vi "DSF.Transceiver.UDP.Rx.Read Datagram.vi"(8 "error in (no error)":errorcluster, 10 "Transfer Group Rx parameters":T1={"Transfers Rx"=[], "max size"=548} {"max size" format="%d bytes"; "Transfers Rx"."timeout" format="%d ms"; "Transfers Rx"."max size" format="%d bytes"}, 11 "UDP Transceiver in":refnum<class "DSF.Transceiver.UDP.lvclass">) -> (0 "error out":errorcluster, 1 "data":string, 2 "Transfer index":i32, 3 "UDP Transceiver out":refnum<class "DSF.Transceiver.UDP.lvclass">)   [LabVIEW 2017, in "DSF.Transceiver.UDP.lvlib" / "DSF.Transceiver.UDP.lvclass"]
uses:
  DSF.Transceiver.UDP.lvclass
  DSF.Transceiver.UDP.Parameters.Transfer Group.Rx.ctl
  DSF.Transceiver.UDP.Parameters.Transfer.Rx.ctl
  DSF.Transceiver.UDP.lvclass/DSF.Transceiver.UDP.ctl
  DSF.Transceiver.UDP.Errors.Rx.Unknown Datagram.vi
  <vilib>/NI/Static Error Handling/VIs/Static Error Handling.Source Buffer.Write.String.vi
  <vilib>/NI/Static Error Handling/VIs/Static Error Handling.Source Buffer.Write.Numeric.Scalar.Base10.vi
  <vilib>/NI/Static Error Handling/VIs/Static Error Handling.Source Buffer.Write.Numeric.Scalar.Base10 (U16).vi
  DSF.Transceiver.UDP.Error.Create.vi
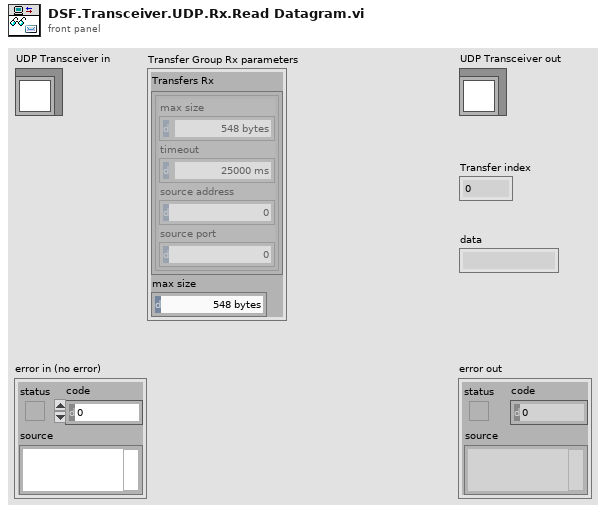
[diagram p1: front panel]
types:
  T1 = typedef "DSF.Transceiver.UDP.lvlib/DSF.Transceiver.UDP.lvclass/DSF.Transceiver.UDP.Parameters.Transfer Group.Rx.ctl" = cluster{"Transfers Rx":T2[], "max size":i32}
  T2 = typedef "DSF.Transceiver.UDP.lvlib/DSF.Transceiver.UDP.lvclass/DSF.Transceiver.UDP.Parameters.Transfer.Rx.ctl" = cluster{"max size":i32, "timeout":i32, "source address":u32, "source port":u16}
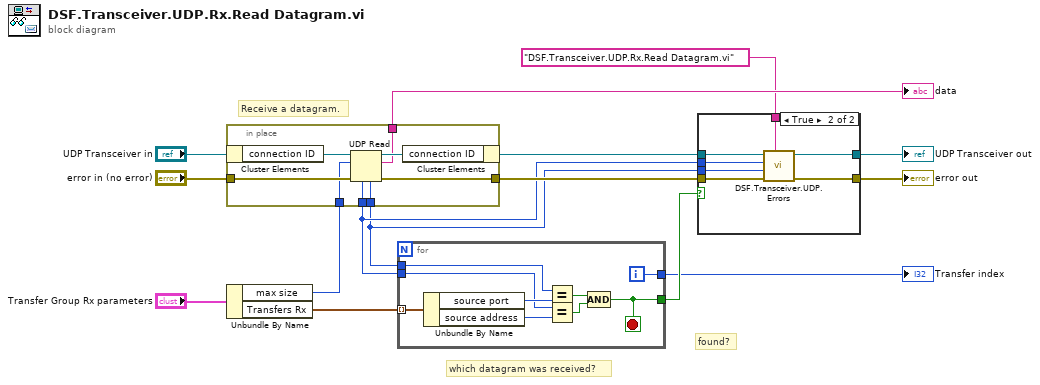
[diagram p0: block diagram]
diagram:
  # "found?"
  # "Receive a datagram."
  # "which datagram was received?"
  n1 = Unbundle By Name("Transfer Group Rx parameters") -> ("max size"=w12:i32, "Transfers Rx"=w11:T2[])
  n2 = in-place {
    in-place-border: "error in (no error)" -> [w23]
    in-place-border: [w21] -> w10
    in-place-border: [w19] -> w6
    in-place-border: [w18] -> w5
    in-place-border: w12 -> [w17]
    in-place-border: [w16] -> w2
    n3 = in-place-cluster #1("UDP Transceiver in") -> ("connection ID"=w20:refnum<k16>)
    n4 = UDP Read(connection ID=w20, max size (548)=w17, 8:w23) -> (data out=w16:string, error out=w21:errorcluster, 3:w22:refnum<k16>, 4:w18:u16, 6:w19:u32)  [unwired: 1 in]
    n5 = in-place-cluster #1("connection ID"=w22) -> (w9:refnum<class "DSF.Transceiver.UDP.lvclass">)
  }
  "data" <- w2
  n6 = for {
    tunnel: w11 -> [w32] mode=indexing
    tunnel: w6 -> [w29]
    tunnel: w5 -> [w28]
    tunnel: [w25] -> w3
    tunnel: [w24] -> w4
    i -> [w25]
    stop <- w24 stop-if-true
    n7 = Unbundle By Name(w32) -> ("source port"=w30:u16, "source address"=w31:u32)
    n8 = Equal?(x=w28, y=w30) -> (x = y?=w26:bool)
    n9 = Equal?(x=w29, y=w31) -> (x = y?=w27:bool)
    n10 = Compound Arithmetic op=AND(w26, w27) -> (w24:bool)
  }
  "Transfer index" <- w3
  n11 = case shown="True" w4 {
    tunnel: w10 -> [w33 w40]
    tunnel: w9 -> [w34 w41]
    tunnel: [w34 w39] -> w8
    tunnel: [w33 w38] -> w7
    tunnel: w6 -> [_ w37]
    tunnel: w5 -> [_ w36]
    tunnel: "DSF.Transceiver.UDP.Rx.Read Datagram.vi" ("source vi name") -> [_ w35]
    frame False {
    }
    frame True {
      n12 = call-poly "DSF.Transceiver.UDP.Errors.vi"("source vi name"=w35, "error in (no error)"=w40, "source port"=w36, "source address"=w37, "UDP Transceiver in"=w41) -> ("error out"=w38:errorcluster, "UDP Transceiver out"=w39:refnum<class "DSF.Transceiver.UDP.lvclass">)  [unwired: 5 in]
    }
  }
  "error out" <- w7
  "UDP Transceiver out" <- w8
